vi "LVFunction_Imop_Pupil_ApplyNeighborExtension.vi"(0 "Pupil in":refnum<class "Pupil.lvclass">, 5 "Pupil OUT":refnum<class "Pupil.lvclass">, 11 "error in (no error)":errorcluster) -> (4 "Pupil out":refnum<class "Pupil.lvclass">, 6 "Pupil OUT 2":refnum<class "Pupil.lvclass">, 15 "error out":errorcluster)   [LabVIEW 2020]
uses:
  Pupil.lvclass
  LVClass_Pupil Read Pupil.vi
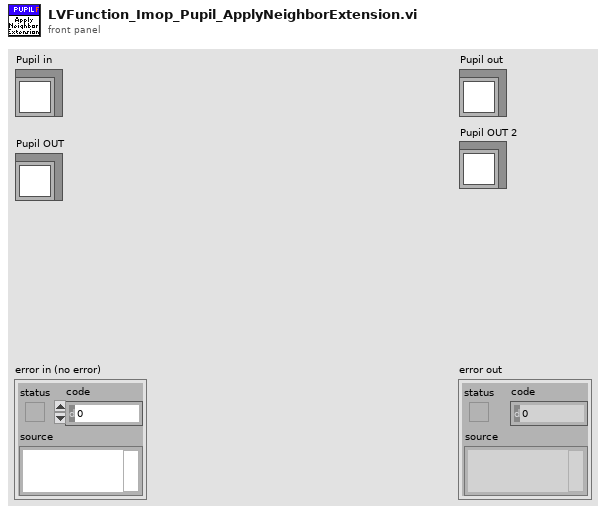
[diagram p1: front panel]
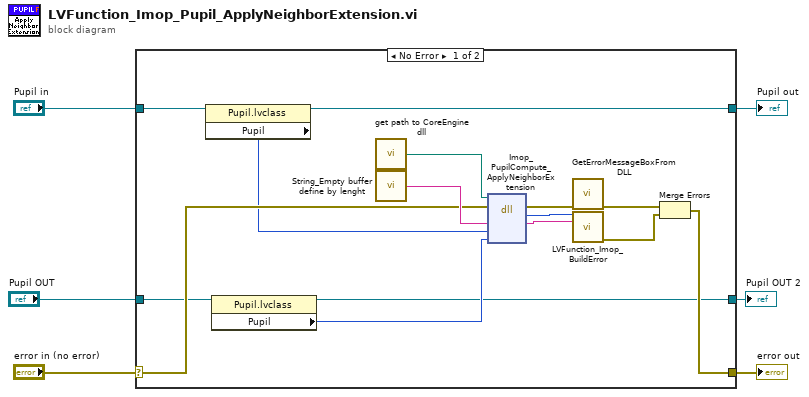
[diagram p0: block diagram]
diagram:
  n1 = case shown="No Error" "error in (no error)" {
    selector: "error in (no error)" -> [w14 w23]
    tunnel: [w13 w23] -> w5
    tunnel: [w8 w22] -> w3
    tunnel: "Pupil in" -> [w9 w22]
    tunnel: "Pupil OUT" -> [w12 _]
    tunnel: [w10 _] -> w1
    frame No Error {
      n2 = property class="Pupil.lvclass"(reference=w9) -> (reference out=w8:refnum<class "Pupil.lvclass">, "Pupil"=w7:i32)  [unwired: 1 in, 1 out]
      n3 = property class="Pupil.lvclass"(reference=w12) -> (reference out=w10:refnum<class "Pupil.lvclass">, "Pupil"=w11:i32)  [unwired: 1 in, 1 out]
      n4 = call "get path to CoreEngine dll.vi"() -> ("path to c_interface_vc100.dll"=w18:path)  [unwired: 12 in, 3 out]
      n5 = call "String_Empty buffer define by lenght.vi"() -> ("Empty buffer"=w21:string)  [unwired: 1 in]
      n6 = dll-call lib="D:/FLE/0.Code/CoreEngine4_Suite/LV2011_interface/DLLs/c_interface_vc100.dll" fn="Imop_PupilCompute_ApplyNeighborExtension"(path in=w18, error in=w14, "message"=w21, "Pupil IN"=w7, "Pupil OUT"=w11) -> (error out=w17:errorcluster, "return type"=w19:i32, "message"=w20:string)  [unwired: 3 in, 1 out]
      n7 = call "GetErrorMessageBoxFromDLL.vi"("error IN"=w17) -> ("error OUT"=w16:errorcluster)  [unwired: 10 in]
      n8 = call "LVFunction_Imop_BuildError.vi"("code"=w19, "String to Prepend to source (\"\")"=w20) -> ("error out"=w15:errorcluster)  [unwired: 13 in]
      n9 = Merge Errors(w16, w15) -> (w13:errorcluster)
    }
    frame Error {
    }
  }
  "error out" <- w5
  "Pupil out" <- w3
  "Pupil OUT 2" <- w1
